vi "EnFlo_Tunnel_Display.vi"() -> ()   [LabVIEW 2013]
uses:
  <vilib>/gmath/NI_Gmath.lvlib
panel:
  out "Lateral profiles":cluster{"Y Axis Current":dbl[], dbl[]}[](graph)
  out "Setpoints":dbl[](array[numeric])
  in  "Subtract Setpoint?":bool
  out "Vert Disp (mm)  @ 14m":dbl
  out "Inlet St Dev":dbl format="%#.3g"
  out "Inlet mapping":dbl[][](graph)=[[0.00729, 0.18153463174730816, 0.17352738437348433, 1.6752433719500537, 8.231465735195274, 17.570357598383207, 23.099772817121426, 25.58386930448374, 25.31727725753219, 24.28926231541072, 18.717383219374323, 10.355253339797807, 2.7760273383248344, 0.3109897541921306, 0.08276881403435009, 0.06197], [0.04411, 0.1361526368018142, 0.04039202183336771, 1.5611636795339547, 8.176972694107874, 17.32000974741714, 24.257541358764026, 25.949153465972987, 26.01802540761648, 25.060373307424115, 18.284750328365213, 8.689831176707928, 2.642937641487066, 0.43219350072447926, -0.019957690739617468, 0.07351], [0.05478, 0.03446320268089581, 0.2086595806581808, 1.6919212249796047, 6.580368005180591, 14.333585185483123, 21.06810094963999, 23.709254571137723, 24.04768940379576, 21.01660820522005, 13.60443428327954, 6.2766496258038735, 1.7988963349022484, 0.2952877651784204, 0.05436788410934033, 0.1022], [0.04013, 0.06419557464541133, 0.2035068586120256, 1.3118741659450193, 4.7061387064566835, 9.009825946069038, 12.927700276268434, 17.003135081884164, 16.83885730812343, 12.902263313363814, 8.246161922417906, 4.035269404379355, 1.329605659745338, 0.24574055091433544, 0.012829784119986217, 0.08755], [0.04404, 0.022691144295571734, 0.19102098261858932, 0.8525411026079828, 2.2353542219792946, 3.966676465246214, 6.305347763088489, 8.17672908183636, 7.7348668140659, 5.703994479070454, 3.8329088824353237, 1.9256956625267279, 0.6611488869641811, 0.20508248283573002, 0.10119553469307395, 0.08441]]
  out "Floor Powers":cluster{"Array":dbl[], dbl[]}(graph)
  in  "Averaging time (mins)":dbl=0.5 format="%.2f"
  out "Ref_2":dbl format="%.3g"
  in  "History in Minutes":dbl
  out "Strat":cluster{dbl[], dbl[]}[](graph)
  out "Des Air Temp":dbl format="%#.2g"
  out "Heat Extraction kW":dbl format="%#.2g"
  out "Av Lab Temp":dbl format="%#.2g"
  out "Av Exit  Temp":dbl format="%#.2g"
  out "Exit Dem Temp":dbl format="%#.2g"
  out "Heat Exchanger Valve %":dbl format="%#.1f"
  out "Delta T":dbl format="%#.2g"
  out "Pump Speed %":dbl format="%#.0f"
  out "Meas Delta P":dbl format="%#.2g"
  out "Desired Delta P":dbl format="%#.2f"
  out "Return Pressure":dbl format="%#.2g"
  out "Supply Pressure":dbl format="%#.2g"
  out "Max Motor Temp":dbl format="%#.1g"
  out "% Speed Tweak":dbl format="%#.2g"
  out "Shaft RPM":dbl format="%#.2g"
  out "K Factor":dbl format="%#.2g"
  out "Tunnel Speed  m/s":dbl format="%.3g"
  out "Uni Chilled water Temp":dbl format="%#.2g"
  out "Mixing Valve %":dbl format="%#.1f"
  out "Dem Temp":dbl
  out "Return Temp":dbl format="%#.2g"
  out "Supply Temp":dbl format="%#.2g"
  out "Floor_Cooling:Enable":bool
  out "Chiller_Pump:Enable":bool
  out "Panel Temps":cluster{"Array":dbl[], dbl[]}[](graph)
  in  "Stop Button":bool
  out "Heaters Enabled":bool
  out "Inlet Heaters":cluster{"yi":dbl[], dbl[]}[](graph)
  # "Chiller Pump Information"
  # "Chilled Water"
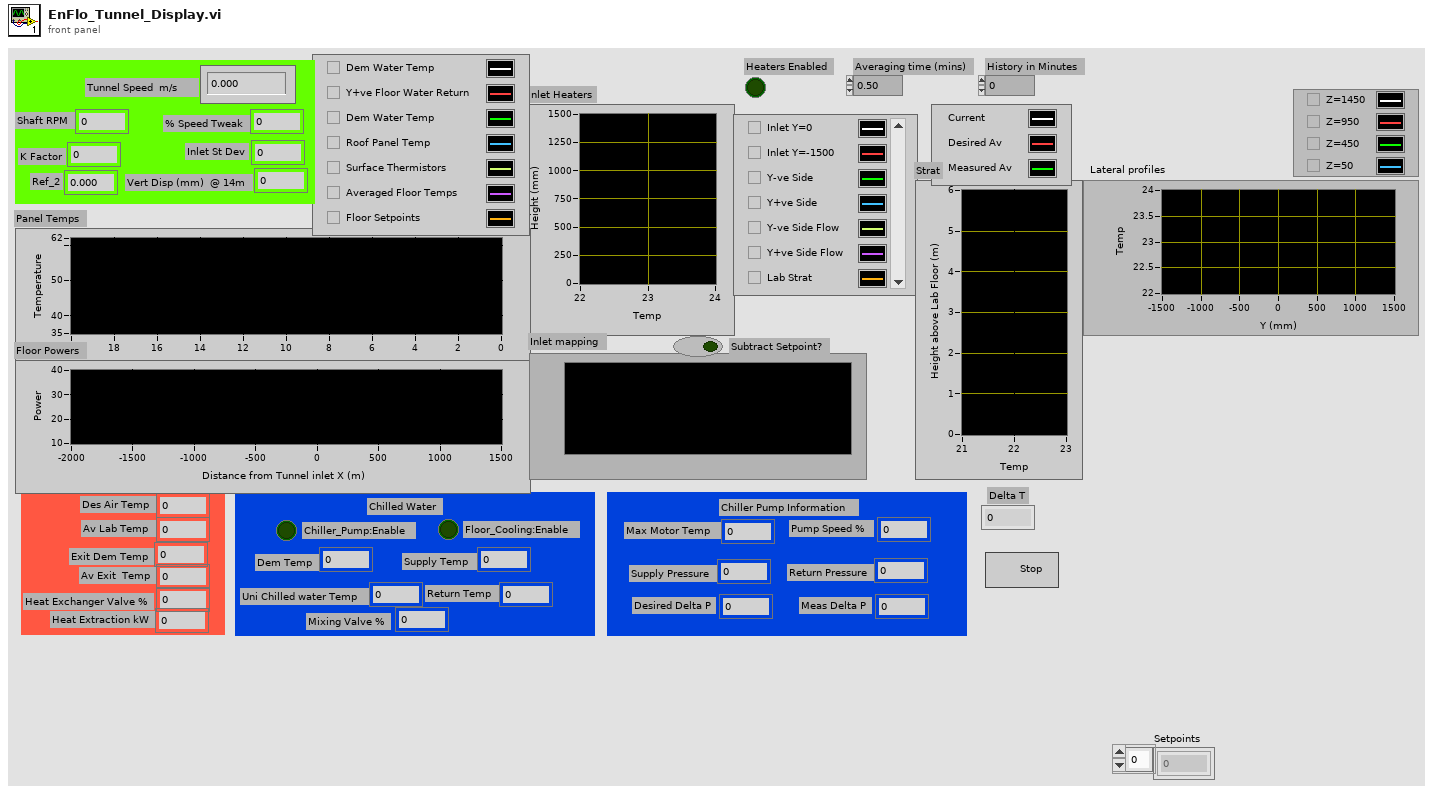
[diagram p1: front panel]
types:
  T1 = cluster{"X Max":dbl, "Y Max ":dbl, "X Scale":cluster{"Xo":dbl, "delta X":dbl}, "Y Scale":cluster{"Xo":dbl, "delta X":dbl}, "X Values":dbl[], "Y Values":dbl[], "Z Max":dbl, "Z Min":dbl}
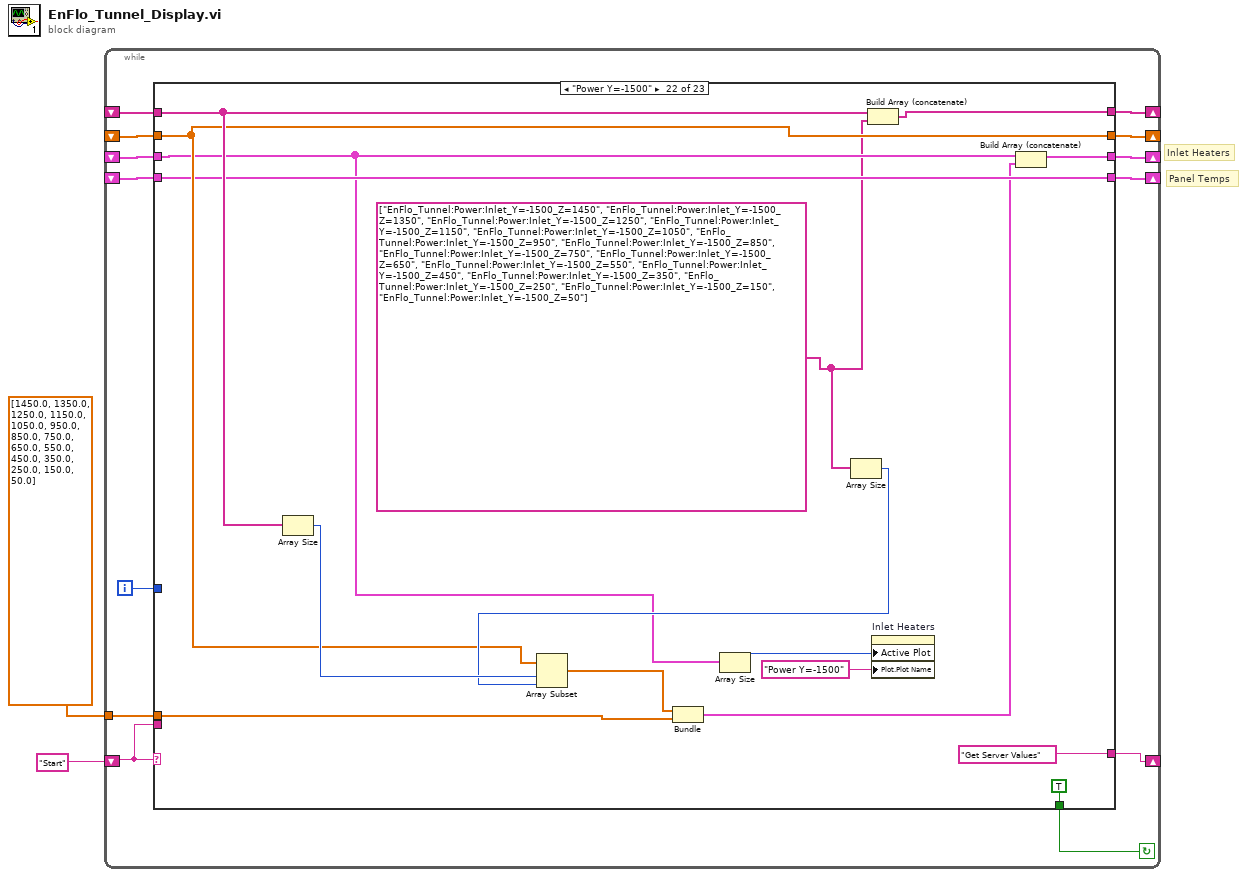
[diagram p0: block diagram]
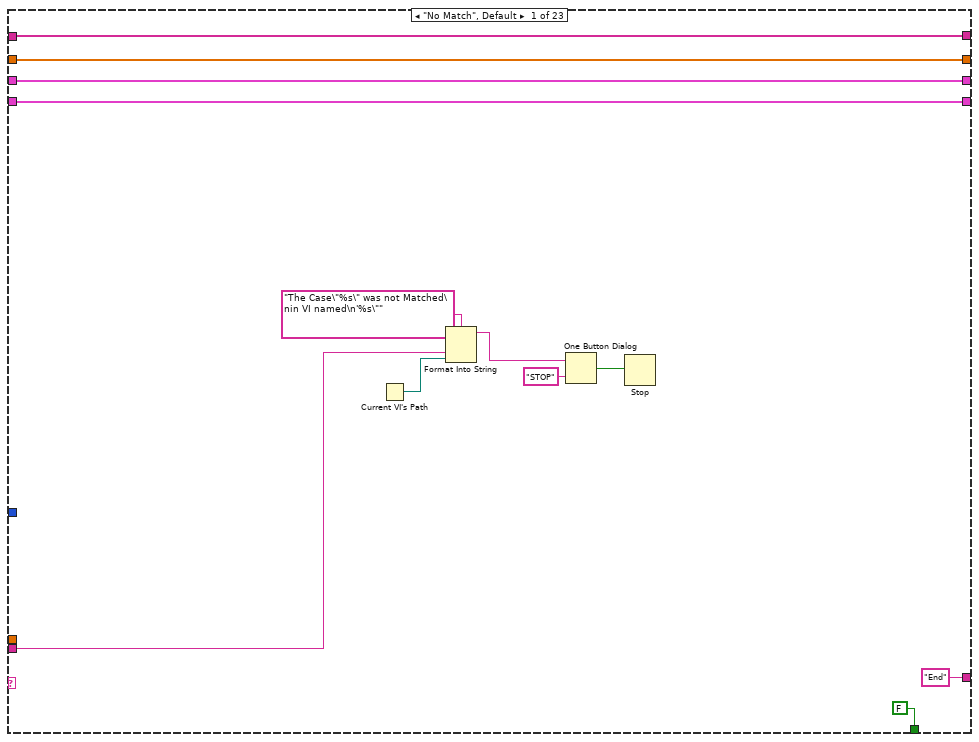
[diagram p2: hidden frame]
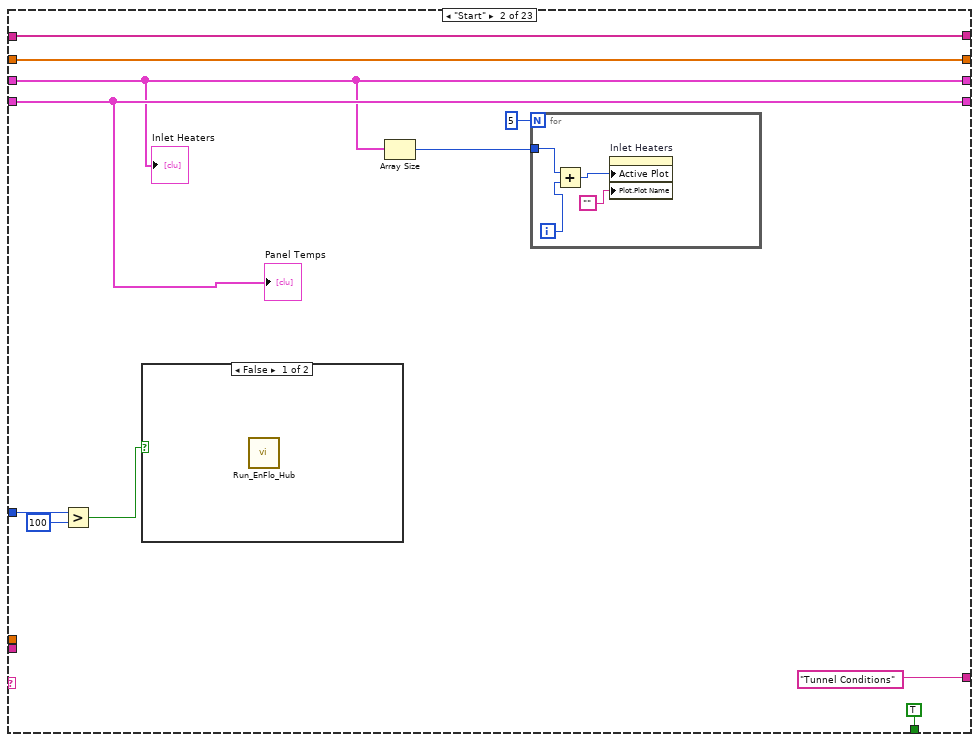
[diagram p3: hidden frame]
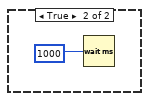
[diagram p4: hidden frame]
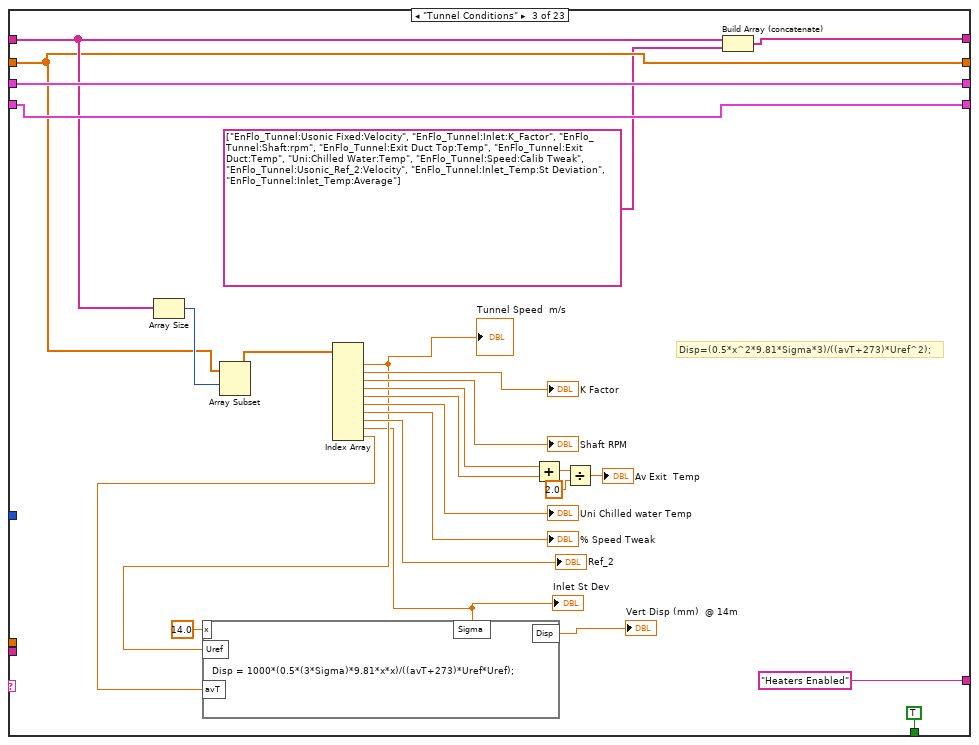
[diagram p5: hidden frame]
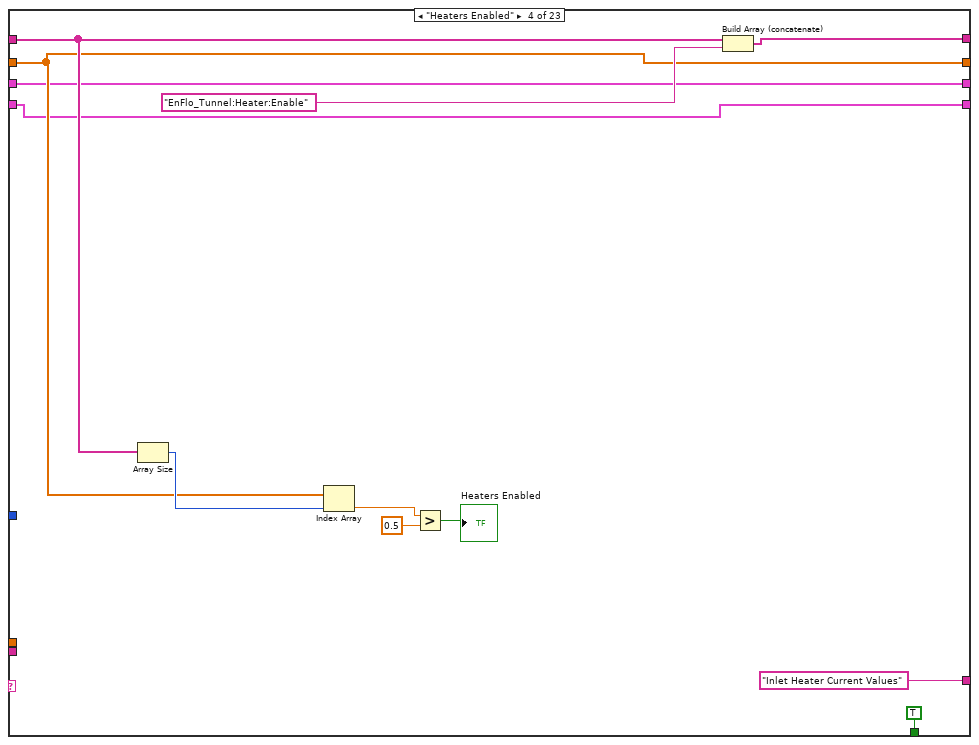
[diagram p6: hidden frame]
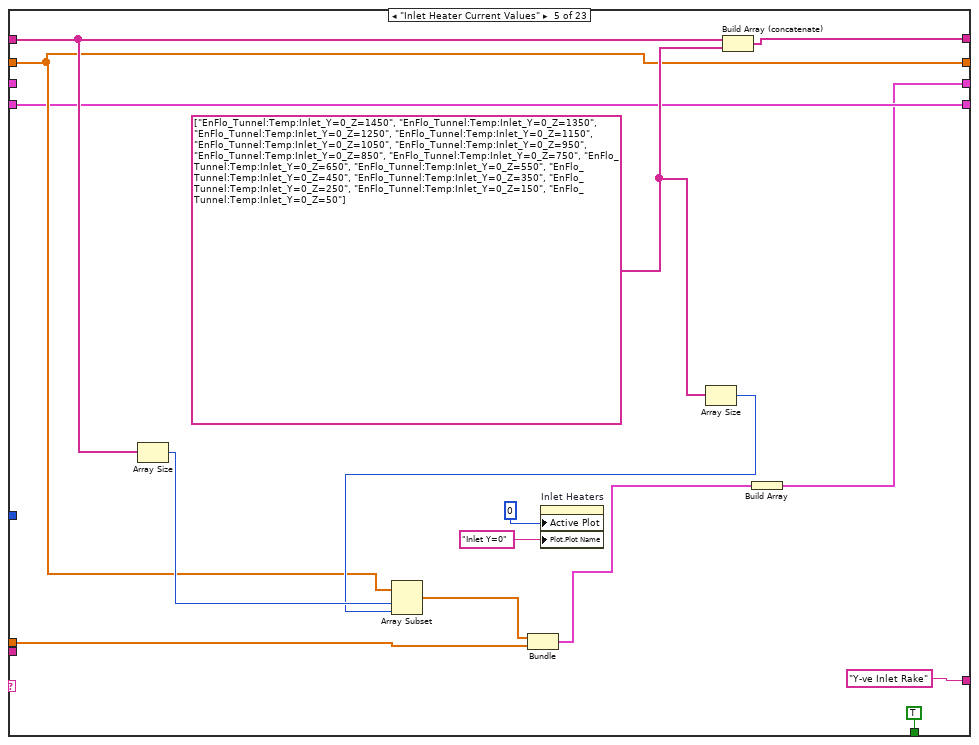
[diagram p7: hidden frame]
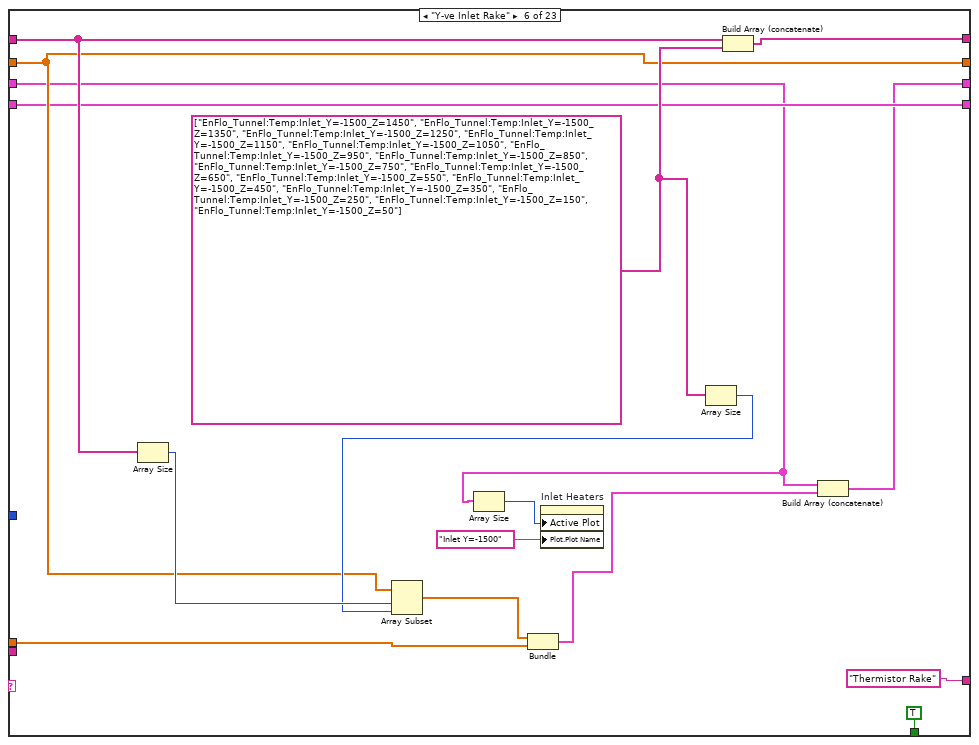
[diagram p8: hidden frame]
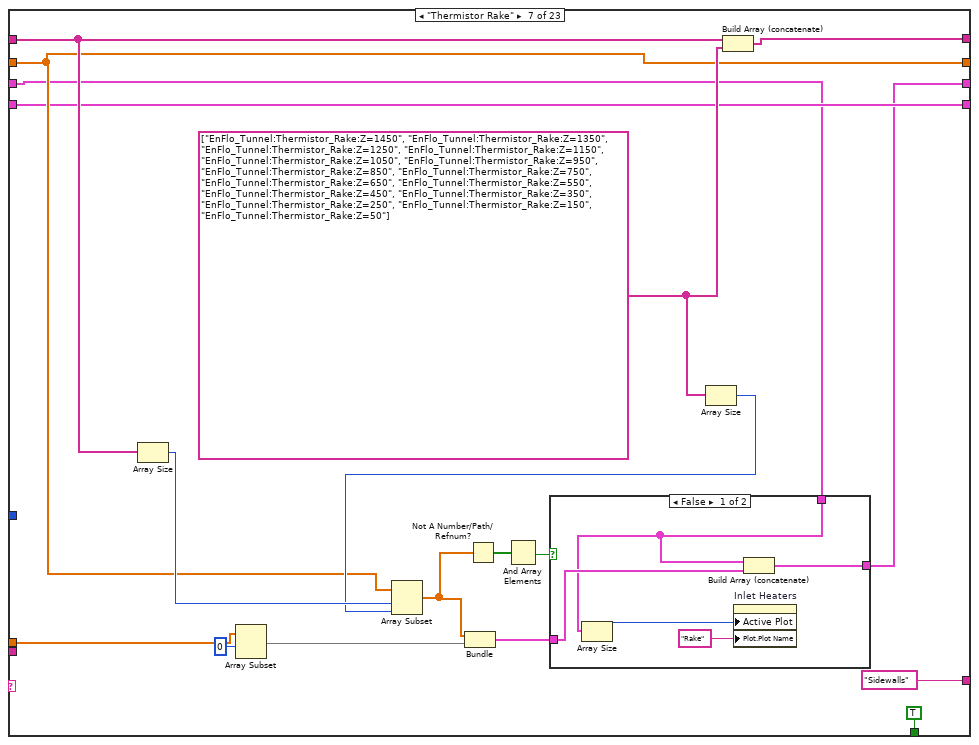
[diagram p9: hidden frame]
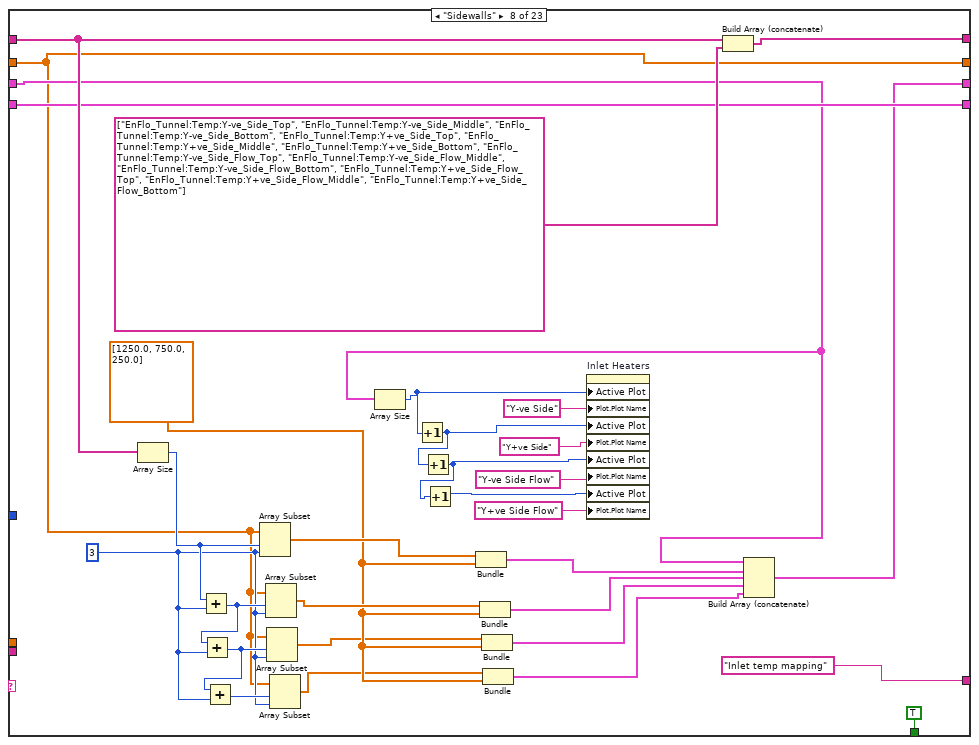
[diagram p11: hidden frame]
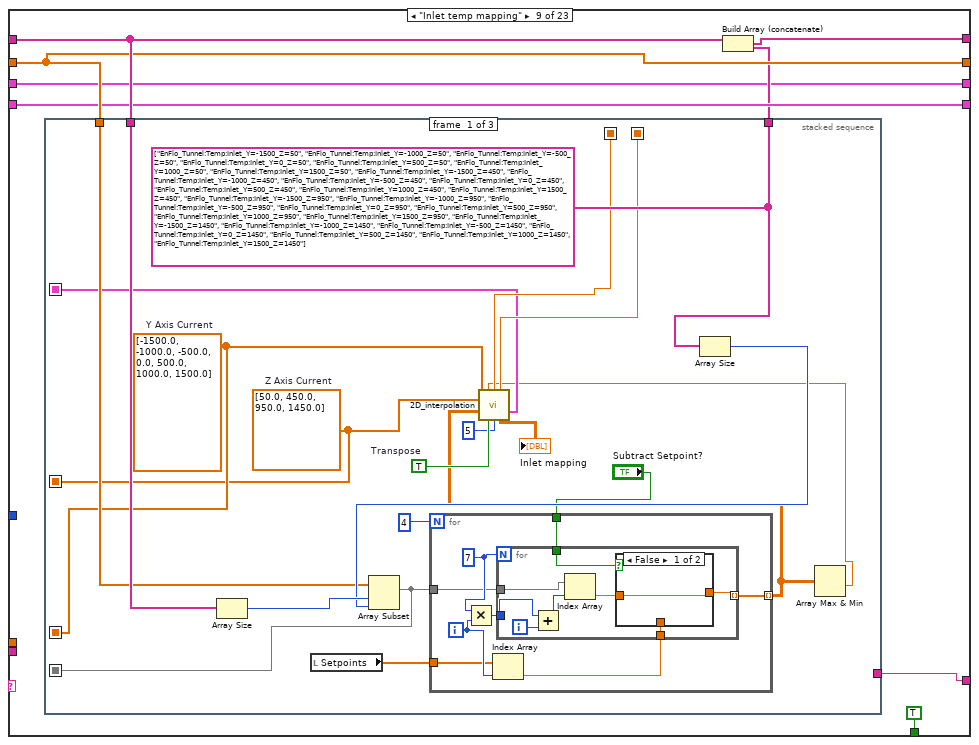
[diagram p12: hidden frame]
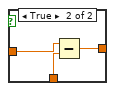
[diagram p13: hidden frame]
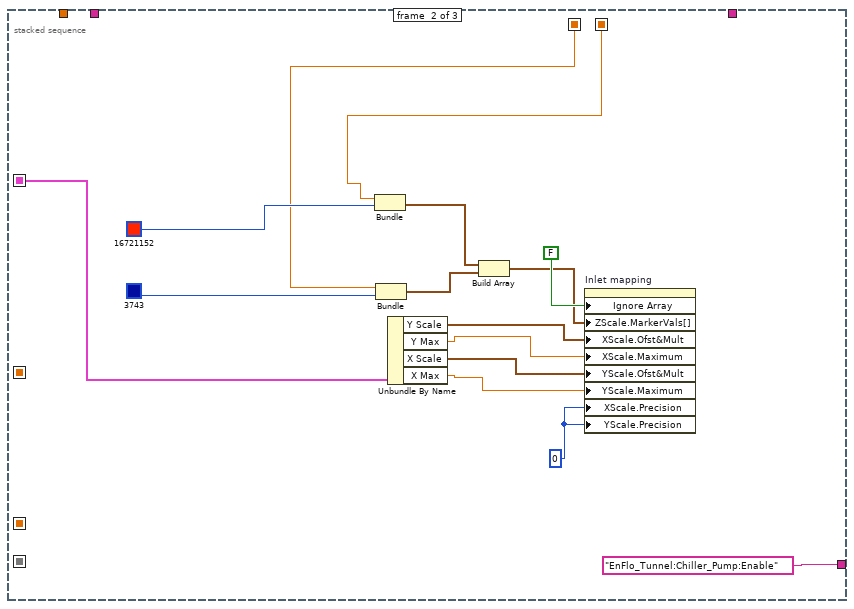
[diagram p14: hidden frame]
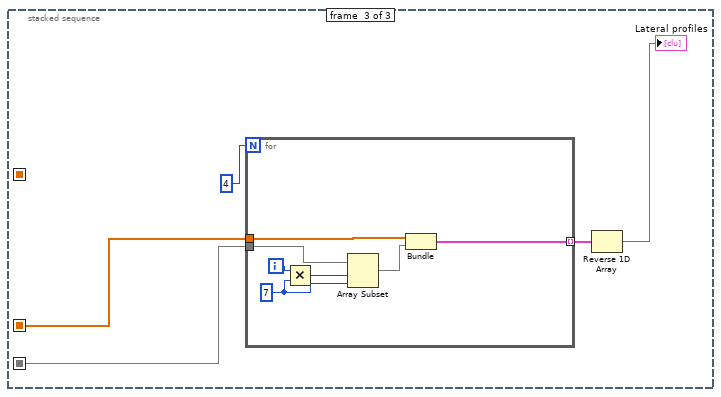
[diagram p15: hidden frame]
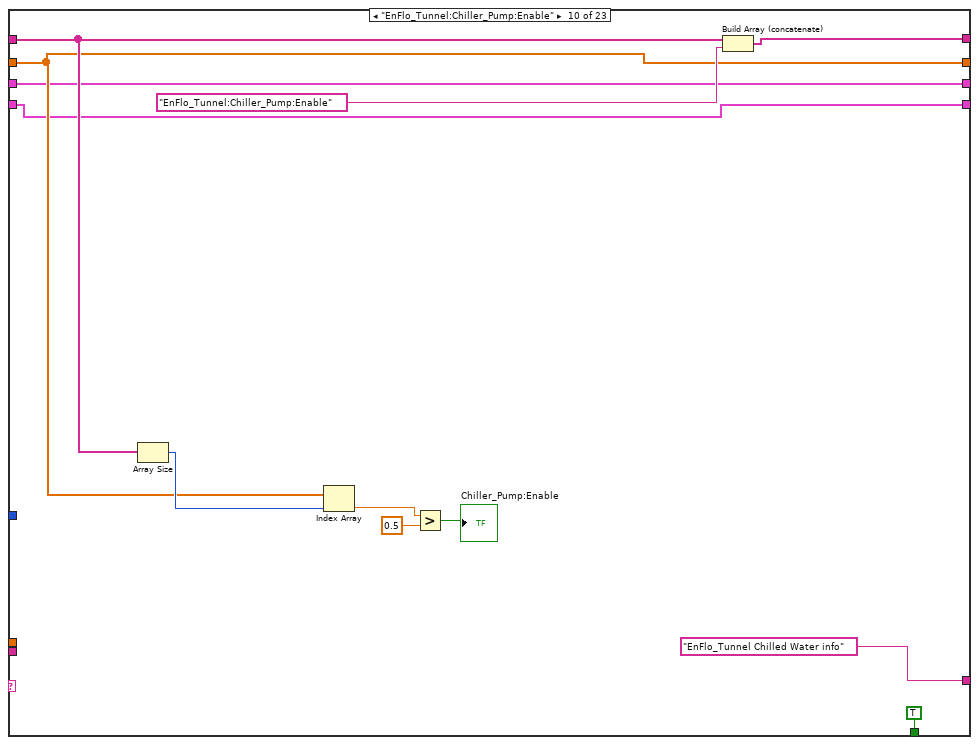
[diagram p16: hidden frame]
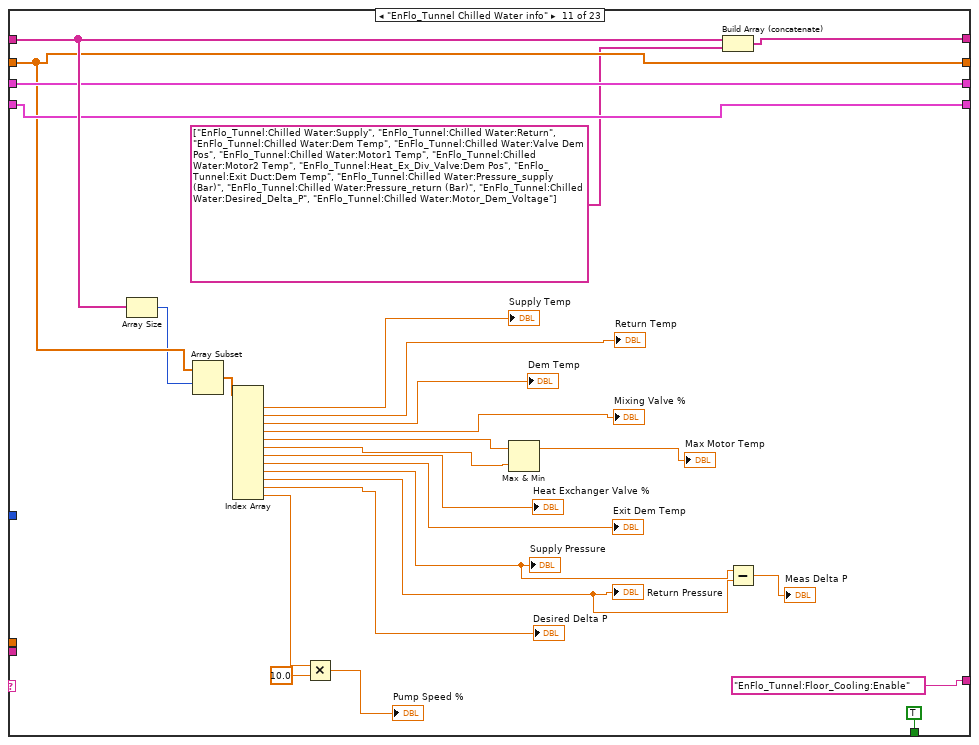
[diagram p17: hidden frame]
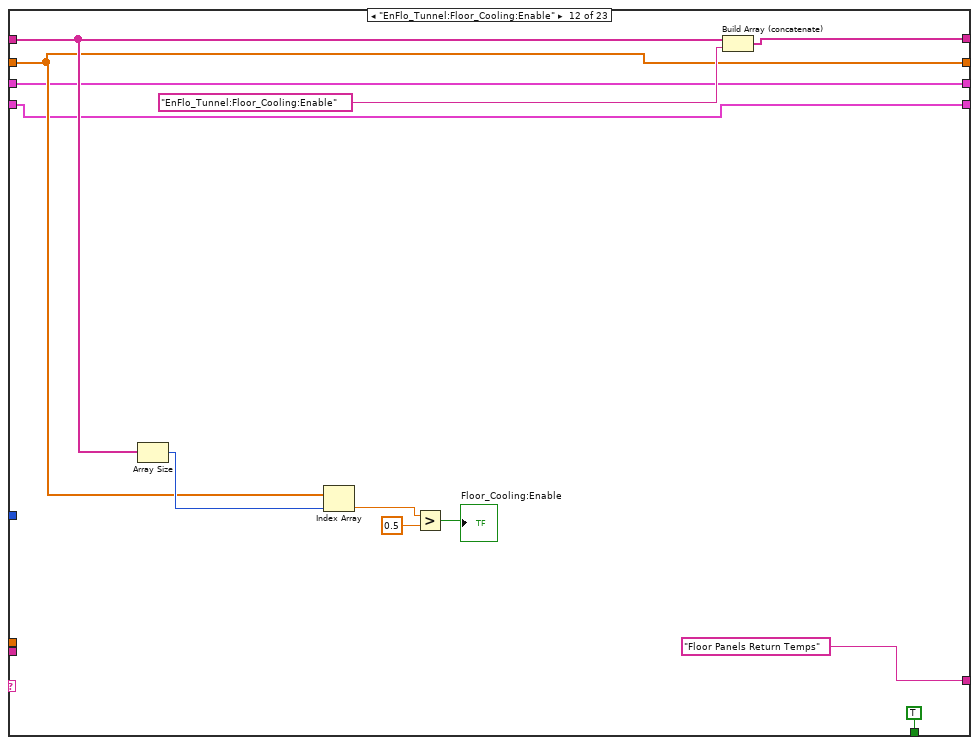
[diagram p18: hidden frame]
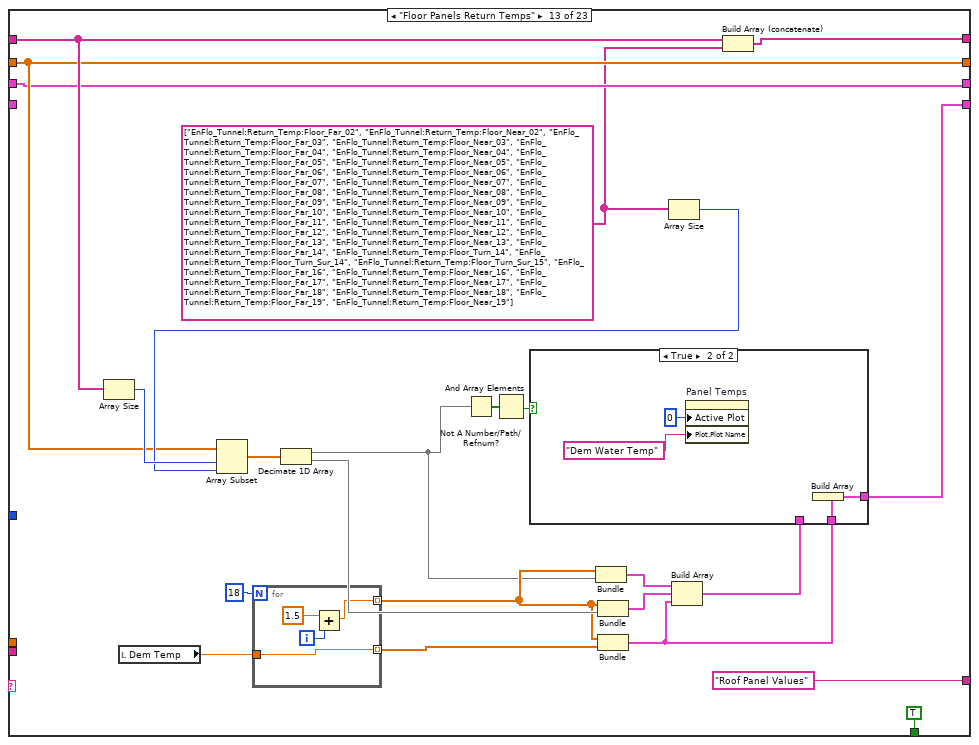
[diagram p19: hidden frame]
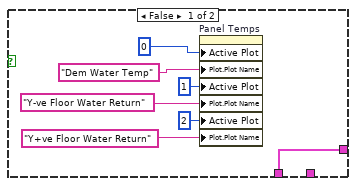
[diagram p20: hidden frame]
diagram:
  # "Panel Temps"
  # "Inlet Heaters"
  n1 = while {
    shift-right: [w13] -> _
    shift-left: "Start" -> [w14]
    shift-right: [w12] -> _
    shift-left: _ -> [w11]
    shift-right: [w9] -> _
    shift-left: _ -> [w10]
    shift-right: [w7] -> _
    shift-left: _ -> [w8]
    shift-right: [w6] -> _
    shift-left: _ -> [w5]
    tunnel: dbl[] [1450.0, 1350.0, 1250.0, 1150.0, 1050.0, 950.0, 850.0, 750.0, 650.0, 550.0, 450.0, 350.0, 250.0, 150.0, 50.0] -> [w3]
    i -> [w4]
    stop <- w15 continue-if-true
    n2 = case shown="\"Power Y=-1500\"" w14 {
      tunnel: [FALSE TRUE TRUE TRUE TRUE TRUE TRUE TRUE TRUE TRUE TRUE TRUE TRUE TRUE TRUE TRUE TRUE TRUE TRUE TRUE TRUE TRUE w500] -> w15
      tunnel: w14 -> [w21 _ _ _ _ _ _ _ _ _ _ _ _ _ _ _ _ _ _ _ _ _ _]
      tunnel: ["End" "Tunnel Conditions" "Heaters Enabled" "Inlet Heater Current Values" "Y-ve Inlet Rake" "Thermistor Rake" "Sidewalls" "Inlet temp mapping" w167 "EnFlo_Tunnel Chilled Water info" "EnFlo_Tunnel:Floor_Cooling:Enable" "Floor Panels Return Temps" "Roof Panel Values" "Floor Surface Panels" "Floor Panel Averages" "Floor Panel Setpoints" "Floor Panel Powers" "Lab Stratification" w398 "Inlet Heater Power Values" "Power Y=-1500" "Get Server Values" "Start"] -> w13
      tunnel: [w19 w37 w66 w78 w93 w109 w127 w164 w173 w251 w277 w289 w311 w340 w354 w368 w382 w395 w431 w456 w475 w491 string[] []] -> w12
      tunnel: w11 -> [w19 w37 w61 w77 w92 w108 w126 w163 w172 w250 w276 w288 w310 w339 w353 w367 w381 w394 w430 w455 w474 w490 w504]
      tunnel: w10 -> [w18 w36 w60 w74 w89 w105 w123 w138 w171 w247 w271 w285 w307 w336 w350 w364 w378 w391 w417 w452 w471 w487 _]
      tunnel: [w18 w36 w60 w74 w89 w105 w123 w138 w171 w247 w271 w285 w307 w336 w350 w364 w378 w391 w417 w452 w471 w487 w503] -> w9
      tunnel: w8 -> [w17 w30 w65 w73 _ w97 w119 w153 w168 w246 w275 w284 w305 w335 w349 w363 w377 w390 w400 w443 w463 w479 w498]
      tunnel: [w17 w30 w65 w73 w82 w100 w120 w159 w168 w246 w275 w284 w305 w335 w349 w363 w377 w390 w421 w450 w467 w483 w498] -> w7
      tunnel: w5 -> [w16 w34 w64 w69 w88 w104 w122 w162 w170 w242 w274 w280 _ w334 w348 w362 w376 w386 w429 w449 w469 w485 w497]
      tunnel: [w16 w34 w64 w69 w88 w104 w122 w162 w170 w242 w274 w280 w292 w333 w347 w361 w375 w386 w429 w449 w469 w485 w497] -> w6
      tunnel: w4 -> [_ w33 _ _ _ _ _ _ _ _ _ _ _ _ _ _ _ _ _ _ _ _ _]
      tunnel: w3 -> [_ _ _ _ w86 w102 w114 _ _ _ _ _ _ _ _ _ _ _ w403 w444 w468 w484 _]
      frame "No Match", Default {
        n3 = Current VI's Path() -> (path=w26:path)
        n4 = Format Into String(format string="The Case\"%s\" was not Matched\nin VI named\n'%s\"" ("Format String"), w21, w26) -> (resulting string=w23:string)  [unwired: 2 in, 1 out]
        n5 = One Button Dialog(message=w23, button name ("OK")="STOP") -> (true=w25:bool)
        n6 = Stop(stop? (T)=w25) -> ()
      }
      frame "Start" {
        n7 = Greater?(x=w33, y=100) -> (0:w31:bool)
        n8 = case shown="False" w31 {
          frame False {
            n9 = call "Run_EnFlo_Hub.vi"() -> ()  [unwired: 8 in]
          }
          frame True {
            n10 = Wait (ms)(milliseconds to wait=u32 1000 ("millisecond timer value")) -> ()  [unwired: 1 out]
          }
        }
        n11 = Array Size(array=w30) -> (size(s)=w28:i32)
        n12 = for {
          N: 5 -> [_]
          tunnel: w28 -> [w42]
          i -> [w41]
          n13 = Add(x=w42, y=w41) -> (x+y=w40:i32)
          n14 = property on="Inlet Heaters" class="XYGraph (strict)"("Active Plot"=w40, "Plot.Plot Name"="") -> ()  [unwired: 2 in, 2 out]
        }
        "Inlet Heaters" <- w30
        "Panel Temps" <- w34
      }
      frame "Tunnel Conditions" {
        # "Disp=(0.5*x^2*9.81*Sigma*3)/((avT+273)*Uref^2);"
        n15 = Array Size(array=w61) -> (size(s)=w63:i32)
        n16 = Array Subset(array=w60, index=w63) -> (w62:dbl[])  [unwired: 1 in]
        n17 = Index Array(array=w62) -> (element #1=w47:dbl, element #2=→"K Factor":dbl, element #3=→"Shaft RPM":dbl, element #4=w53:dbl, element #5=w52:dbl, element #6=→"Uni Chilled water Temp":dbl, element #7=→"% Speed Tweak":dbl, element #8=→"Ref_2":dbl, element #9=w46:dbl, element #10=w45:dbl)  [unwired: 10 in]
        "Tunnel Speed  m/s" <- w47
        "Inlet St Dev" <- w46
        n18 = formula code="Disp = 1000*(0.5*(3*Sigma)*9.81*x*x)/((avT+273)*Uref*Uref);"("x"=14.0 ("input variable"), "Uref"=w47, "Sigma"=w46, "avT"=w45) -> ("Disp"=→"Vert Disp (mm)  @ 14m":dbl)
        n19 = Add(x=w53, y=w52) -> (x+y=w57:dbl)
        n20 = Divide(x=w57, y=2.0) -> (x/y=→"Av Exit  Temp":dbl)
        n21 = Build Array (concatenate)(w61, string[] ["EnFlo_Tunnel:Usonic Fixed:Velocity", "EnFlo_Tunnel:Inlet:K_Factor", "EnFlo_Tunnel:Shaft:rpm", "EnFlo_Tunnel:Exit Duct Top:Temp", "EnFlo_Tunnel:Exit Duct:Temp", "Uni:Chilled Water:Temp", "EnFlo_Tunnel:Speed:Calib Tweak", "EnFlo_Tunnel:Usonic_Ref_2:Velocity", "EnFlo_Tunnel:Inlet_Temp:St Deviation", "EnFlo_Tunnel:Inlet_Temp:Average"] ("subarray")) -> (w66:string[])
      }
      frame "Heaters Enabled" {
        n22 = Array Size(array=w77) -> (size(s)=w75:i32)
        n23 = Index Array(array=w74, index=w75) -> (element=w72:dbl)
        n24 = Greater?(x=w72, y=0.5) -> (0:→"Heaters Enabled":bool)
        n25 = Build Array (concatenate)(w77, "EnFlo_Tunnel:Heater:Enable" ("Ch Name")) -> (w78:string[])
      }
      frame "Inlet Heater Current Values" {
        w94 = string[] ["EnFlo_Tunnel:Temp:Inlet_Y=0_Z=1450", "EnFlo_Tunnel:Temp:Inlet_Y=0_Z=1350", "EnFlo_Tunnel:Temp:Inlet_Y=0_Z=1250", "EnFlo_Tunnel:Temp:Inlet_Y=0_Z=1150", "EnFlo_Tunnel:Temp:Inlet_Y=0_Z=1050", "EnFlo_Tunnel:Temp:Inlet_Y=0_Z=950", "EnFlo_Tunnel:Temp:Inlet_Y=0_Z=850", "EnFlo_Tunnel:Temp:Inlet_Y=0_Z=750", "EnFlo_Tunnel:Temp:Inlet_Y=0_Z=650", "EnFlo_Tunnel:Temp:Inlet_Y=0_Z=550", "EnFlo_Tunnel:Temp:Inlet_Y=0_Z=450", "EnFlo_Tunnel:Temp:Inlet_Y=0_Z=350", "EnFlo_Tunnel:Temp:Inlet_Y=0_Z=250", "EnFlo_Tunnel:Temp:Inlet_Y=0_Z=150", "EnFlo_Tunnel:Temp:Inlet_Y=0_Z=50"] ("subarray")
        n26 = Array Size(array=w92) -> (size(s)=w91:i32)
        n27 = property on="Inlet Heaters" class="XYGraph (strict)"("Active Plot"=u32 0, "Plot.Plot Name"="Inlet Y=0") -> ()  [unwired: 2 in, 2 out]
        n28 = Array Size(array=w94) -> (size(s)=w90:i32)
        n29 = Array Subset(array=w89, index=w91, length=w90) -> (w87:dbl[])
        n30 = Bundle(w87, w86) -> (w83:cluster{dbl[], dbl[]})  [unwired: 1 in]
        n31 = Build Array (concatenate)(w92, w94) -> (w93:string[])
        n32 = Build Array(w83) -> (w82:cluster{dbl[], dbl[]}[])
      }
      frame "Y-ve Inlet Rake" {
        w110 = string[] ["EnFlo_Tunnel:Temp:Inlet_Y=-1500_Z=1450", "EnFlo_Tunnel:Temp:Inlet_Y=-1500_Z=1350", "EnFlo_Tunnel:Temp:Inlet_Y=-1500_Z=1250", "EnFlo_Tunnel:Temp:Inlet_Y=-1500_Z=1150", "EnFlo_Tunnel:Temp:Inlet_Y=-1500_Z=1050", "EnFlo_Tunnel:Temp:Inlet_Y=-1500_Z=950", "EnFlo_Tunnel:Temp:Inlet_Y=-1500_Z=850", "EnFlo_Tunnel:Temp:Inlet_Y=-1500_Z=750", "EnFlo_Tunnel:Temp:Inlet_Y=-1500_Z=650", "EnFlo_Tunnel:Temp:Inlet_Y=-1500_Z=550", "EnFlo_Tunnel:Temp:Inlet_Y=-1500_Z=450", "EnFlo_Tunnel:Temp:Inlet_Y=-1500_Z=350", "EnFlo_Tunnel:Temp:Inlet_Y=-1500_Z=250", "EnFlo_Tunnel:Temp:Inlet_Y=-1500_Z=150", "EnFlo_Tunnel:Temp:Inlet_Y=-1500_Z=50"] ("subarray")
        n33 = Array Size(array=w108) -> (size(s)=w107:i32)
        n34 = Array Size(array=w97) -> (size(s)=w96:i32)
        n35 = property on="Inlet Heaters" class="XYGraph (strict)"("Active Plot"=w96, "Plot.Plot Name"="Inlet Y=-1500") -> ()  [unwired: 2 in, 2 out]
        n36 = Array Size(array=w110) -> (size(s)=w106:i32)
        n37 = Array Subset(array=w105, index=w107, length=w106) -> (w103:dbl[])
        n38 = Bundle(w103, w102) -> (w98:cluster{dbl[], dbl[]})  [unwired: 1 in]
        n39 = Build Array (concatenate)(w108, w110) -> (w109:string[])
        n40 = Build Array (concatenate)(w97, w98) -> (w100:cluster{"yi":dbl[], dbl[]}[])
      }
      frame "Thermistor Rake" {
        w128 = string[] ["EnFlo_Tunnel:Thermistor_Rake:Z=1450", "EnFlo_Tunnel:Thermistor_Rake:Z=1350", "EnFlo_Tunnel:Thermistor_Rake:Z=1250", "EnFlo_Tunnel:Thermistor_Rake:Z=1150", "EnFlo_Tunnel:Thermistor_Rake:Z=1050", "EnFlo_Tunnel:Thermistor_Rake:Z=950", "EnFlo_Tunnel:Thermistor_Rake:Z=850", "EnFlo_Tunnel:Thermistor_Rake:Z=750", "EnFlo_Tunnel:Thermistor_Rake:Z=650", "EnFlo_Tunnel:Thermistor_Rake:Z=550", "EnFlo_Tunnel:Thermistor_Rake:Z=450", "EnFlo_Tunnel:Thermistor_Rake:Z=350", "EnFlo_Tunnel:Thermistor_Rake:Z=250", "EnFlo_Tunnel:Thermistor_Rake:Z=150", "EnFlo_Tunnel:Thermistor_Rake:Z=50"] ("subarray")
        n41 = Array Size(array=w126) -> (size(s)=w125:i32)
        n42 = Array Subset(array=w114, index=0) -> (w112:dbl[])  [unwired: 1 in]
        n43 = Array Size(array=w128) -> (size(s)=w124:i32)
        n44 = Array Subset(array=w123, index=w125, length=w124) -> (w118:dbl[])
        n45 = Bundle(w118, w112) -> (w115:cluster{dbl[], dbl[]})  [unwired: 1 in]
        n46 = Not A Number/Path/Refnum?(number/path/refnum=w118) -> (NaN/Path/Refnum?=w117:bool[])
        n47 = And Array Elements(Boolean array=w117) -> (logical AND=w116:bool)
        n48 = case shown="False" w116 {
          tunnel: [w134 w135] -> w120
          tunnel: w119 -> [w130 w135]
          tunnel: w115 -> [w133 _]
          frame False {
            n49 = Array Size(array=w130) -> (size(s)=w131:i32)
            n50 = property on="Inlet Heaters" class="XYGraph (strict)"("Active Plot"=w131, "Plot.Plot Name"="Rake") -> ()  [unwired: 2 in, 2 out]
            n51 = Build Array (concatenate)(w130, w133) -> (w134:cluster{"yi":dbl[], dbl[]}[])
          }
          frame True {
          }
        }
        n52 = Build Array (concatenate)(w126, w128) -> (w127:string[])
      }
      frame "Sidewalls" {
        w141 = dbl[] [1250.0, 750.0, 250.0]
        w142 = 3 ("length")
        n53 = Array Size(array=w163) -> (size(s)=w158:i32)
        n54 = Add(x=w158, y=w142) -> (x+y=w144:i32)
        n55 = Add(x=w144, y=w142) -> (x+y=w143:i32)
        n56 = Add(x=w143, y=w142) -> (x+y=w145:i32)
        n57 = Array Subset(array=w138, index=w158, length=w142) -> (w157:dbl[])
        n58 = Array Subset(array=w138, index=w144, length=w142) -> (w156:dbl[])
        n59 = Array Subset(array=w138, index=w143, length=w142) -> (w140:dbl[])
        n60 = Array Subset(array=w138, index=w145, length=w142) -> (w139:dbl[])
        n61 = Array Size(array=w153) -> (size(s)=w151:i32)
        n62 = Increment(x=w151) -> (x+1=w148:i32)
        n63 = Increment(x=w148) -> (x+1=w146:i32)
        n64 = Increment(x=w146) -> (x+1=w147:i32)
        n65 = Bundle(w157, w141) -> (w160:cluster{dbl[], dbl[]})  [unwired: 1 in]
        n66 = Bundle(w156, w141) -> (w155:cluster{dbl[], dbl[]})  [unwired: 1 in]
        n67 = Bundle(w140, w141) -> (w137:cluster{dbl[], dbl[]})  [unwired: 1 in]
        n68 = Bundle(w139, w141) -> (w136:cluster{dbl[], dbl[]})  [unwired: 1 in]
        n69 = property on="Inlet Heaters" class="XYGraph (strict)"("Active Plot"=w151, "Plot.Plot Name"="Y-ve Side", "Active Plot"=w148, "Plot.Plot Name"="Y+ve Side", "Active Plot"=w146, "Plot.Plot Name"="Y-ve Side Flow", "Active Plot"=w147, "Plot.Plot Name"="Y+ve Side Flow") -> ()  [unwired: 2 in, 2 out]
        n70 = Build Array (concatenate)(w163, string[] ["EnFlo_Tunnel:Temp:Y-ve_Side_Top", "EnFlo_Tunnel:Temp:Y-ve_Side_Middle", "EnFlo_Tunnel:Temp:Y-ve_Side_Bottom", "EnFlo_Tunnel:Temp:Y+ve_Side_Top", "EnFlo_Tunnel:Temp:Y+ve_Side_Middle", "EnFlo_Tunnel:Temp:Y+ve_Side_Bottom", "EnFlo_Tunnel:Temp:Y-ve_Side_Flow_Top", "EnFlo_Tunnel:Temp:Y-ve_Side_Flow_Middle", "EnFlo_Tunnel:Temp:Y-ve_Side_Flow_Bottom", "EnFlo_Tunnel:Temp:Y+ve_Side_Flow_Top", "EnFlo_Tunnel:Temp:Y+ve_Side_Flow_Middle", "EnFlo_Tunnel:Temp:Y+ve_Side_Flow_Bottom"] ("subarray")) -> (w164:string[])
        n71 = Build Array (concatenate)(w153, w160, w155, w137, w136) -> (w159:cluster{"yi":dbl[], dbl[]}[])
      }
      frame "Inlet temp mapping" {
        n72 = stacked-sequence {
          seq-local: [w185 _ _] -> [_ w222 _]
          seq-local: [w184 _ _] -> [_ w223 _]
          seq-local: [w183 _ _] -> [_ w218 _]
          seq-local: [w177 _ _] -> [_ _ w232]
          seq-local: [w176 _ _] -> [_ _ w233]
          seq-local: [w175 _ _] -> [_ _ _]
          tunnel: w172 -> [w193 _ _]
          tunnel: w171 -> [w190 _ _]
          tunnel: [w189 _ _] -> w169
          tunnel: [_ "EnFlo_Tunnel:Chiller_Pump:Enable" _] -> w167
          frame #0 {
            w187 = TRUE  # Transpose
            w175 = dbl[] [50.0, 450.0, 950.0, 1450.0]  # Z Axis Current
            w176 = dbl[] [-1500.0, -1000.0, -500.0, 0.0, 500.0, 1000.0, 1500.0]  # Y Axis Current
            w189 = string[] ["EnFlo_Tunnel:Temp:Inlet_Y=-1500_Z=50", "EnFlo_Tunnel:Temp:Inlet_Y=-1000_Z=50", "EnFlo_Tunnel:Temp:Inlet_Y=-500_Z=50", "EnFlo_Tunnel:Temp:Inlet_Y=0_Z=50", "EnFlo_Tunnel:Temp:Inlet_Y=500_Z=50", "EnFlo_Tunnel:Temp:Inlet_Y=1000_Z=50", "EnFlo_Tunnel:Temp:Inlet_Y=1500_Z=50", "EnFlo_Tunnel:Temp:Inlet_Y=-1500_Z=450", "EnFlo_Tunnel:Temp:Inlet_Y=-1000_Z=450", "EnFlo_Tunnel:Temp:Inlet_Y=-500_Z=450", "EnFlo_Tunnel:Temp:Inlet_Y=0_Z=450", "EnFlo_Tunnel:Temp:Inlet_Y=500_Z=450", "EnFlo_Tunnel:Temp:Inlet_Y=1000_Z=450", "EnFlo_Tunnel:Temp:Inlet_Y=1500_Z=450", "EnFlo_Tunnel:Temp:Inlet_Y=-1500_Z=950", "EnFlo_Tunnel:Temp:Inlet_Y=-1000_Z=950", "EnFlo_Tunnel:Temp:Inlet_Y=-500_Z=950", "EnFlo_Tunnel:Temp:Inlet_Y=0_Z=950", "EnFlo_Tunnel:Temp:Inlet_Y=500_Z=950", "EnFlo_Tunnel:Temp:Inlet_Y=1000_Z=950", "EnFlo_Tunnel:Temp:Inlet_Y=1500_Z=950", "EnFlo_Tunnel:Temp:Inlet_Y=-1500_Z=1450", "EnFlo_Tunnel:Temp:Inlet_Y=-1000_Z=1450", "EnFlo_Tunnel:Temp:Inlet_Y=-500_Z=1450", "EnFlo_Tunnel:Temp:Inlet_Y=0_Z=1450", "EnFlo_Tunnel:Temp:Inlet_Y=500_Z=1450", "EnFlo_Tunnel:Temp:Inlet_Y=1000_Z=1450", "EnFlo_Tunnel:Temp:Inlet_Y=1500_Z=1450"] ("subarray")
            n73 = Array Size(array=w193) -> (size(s)=w192:i32)
            n74 = local read "Setpoints"() -> (w181:dbl[])
            n75 = Array Size(array=w189) -> (size(s)=w191:i32)
            n76 = Array Subset(array=w190, index=w192, length=w191) -> (w177:dbl[])
            n77 = for {
              N: 4 -> [_]
              tunnel: [w199] -> w179 mode=indexing
              tunnel: w181 -> [w197]
              tunnel: "Subtract Setpoint?" -> [w196]
              tunnel: w177 -> [w194]
              i -> [w198]
              w201 = 7
              n78 = Multiply(x=w201, y=w198) -> (x*y=w200:i32)
              n79 = Index Array(array=w197, index=w198) -> (element=w195:dbl)
              n80 = for {
                N: w201 -> [_]
                tunnel: w200 -> [w208]
                tunnel: w194 -> [w206]
                tunnel: [w202] -> w199 mode=indexing
                tunnel: w196 -> [w205]
                tunnel: w195 -> [w203]
                i -> [w209]
                n81 = Add(x=w208, y=w209) -> (x+y=w207:i32)
                n82 = Index Array(array=w206, index=w207) -> (element=w204:dbl)
                n83 = case shown="False" w205 {
                  tunnel: w204 -> [w210 w213]
                  tunnel: w203 -> [_ w212]
                  tunnel: [w210 w211] -> w202
                  frame False {
                  }
                  frame True {
                    n84 = Subtract(x=w213, y=w212) -> (x-y=w211:dbl)
                  }
                }
              }
            }
            n85 = Array Max & Min(array=w179) -> (min value=w178:dbl)  [unwired: 3 out]
            n86 = call "2D_interpolation.vi"("X Axis Current"=w176, "Min Z Value In"=w178, "Y axis Current"=w175, "Plot In"=w179, "Transpose"=w187, "Point Size"=5) -> ("min Z value"=w185:dbl, "max Z value"=w184:dbl, "Axis info"=w183:T1, "Plot Out"=→"Inlet mapping":dbl[][])  [unwired: 2 in, 4 out]
          }
          frame #1 {
            w219 = u8 0 ("X Scale.Display Format:Precision")
            n87 = Bundle("max Z value"=w223, u32 16721152) -> (w226:cluster{"max Z value":dbl, u32})  [unwired: 1 out]
            n88 = Bundle("min Z value"=w222, u32 3743) -> (w227:cluster{"min Z value":dbl, u32})  [unwired: 1 out]
            n89 = Unbundle By Name(w218) -> ("Y Scale"=w217:cluster{"Xo":dbl, "delta X":dbl}, "Y Max"=w216:dbl, "X Scale"=w215:cluster{"Xo":dbl, "delta X":dbl}, "X Max"=w214:dbl)
            n90 = Build Array(w226, w227) -> (w220:cluster{"min Z value":dbl, u32}[])
            n91 = property on="Inlet mapping" class="IntGraph (strict)"("Ignore Array"=FALSE, "ZScale.MarkerVals[]"=w220, "XScale.Ofst&Mult"=w217, "XScale.Maximum"=w216, "YScale.Ofst&Mult"=w215, "YScale.Maximum"=w214, "XScale.Precision"=w219, "YScale.Precision"=w219) -> ()  [unwired: 2 in, 2 out]
          }
          frame #2 {
            n92 = for {
              N: 4 -> [_]
              tunnel: w233 -> [w240]
              tunnel: w232 -> [w239]
              tunnel: [w234] -> w230 mode=indexing
              i -> [w236]
              w238 = 7 ("length")
              n93 = Multiply(x=w236, y=w238) -> (x*y=w237:i32)
              n94 = Array Subset(array=w239, index=w237, length=w238) -> (w235:dbl[])
              n95 = Bundle("Y Axis Current"=w240, w235) -> (w234:cluster{"Y Axis Current":dbl[], dbl[]})  [unwired: 1 in]
            }
            n96 = Reverse 1D Array(array=w230) -> (reversed array=→"Lateral profiles":cluster{"Y Axis Current":dbl[], dbl[]}[])
          }
        }
        n97 = Build Array (concatenate)(w172, w169) -> (w173:string[])
      }
      frame "EnFlo_Tunnel:Chiller_Pump:Enable" {
        n98 = Array Size(array=w250) -> (size(s)=w248:i32)
        n99 = Index Array(array=w247, index=w248) -> (element=w245:dbl)
        n100 = Greater?(x=w245, y=0.5) -> (0:→"Chiller_Pump:Enable":bool)
        n101 = Build Array (concatenate)(w250, "EnFlo_Tunnel:Chiller_Pump:Enable" ("Ch Name")) -> (w251:string[])
      }
      frame "EnFlo_Tunnel Chilled Water info" {
        n102 = Array Size(array=w276) -> (size(s)=w270:i32)
        n103 = Array Subset(array=w271, index=w270) -> (w269:dbl[])  [unwired: 1 in]
        n104 = Index Array(array=w269) -> (element #1=→"Supply Temp":dbl, element #2=→"Return Temp":dbl, element #3=→"Dem Temp":dbl, element #4=→"Mixing Valve %":dbl, element #5=w256:dbl, element #6=w255:dbl, element #7=→"Heat Exchanger Valve %":dbl, element #8=→"Exit Dem Temp":dbl, element #9=w261:dbl, element #10=w260:dbl, element #11=→"Desired Delta P":dbl, element #12=w253:dbl)  [unwired: 12 in]
        "Supply Pressure" <- w261
        "Return Pressure" <- w260
        n105 = Multiply(x=w253, y=10.0) -> (x*y=→"Pump Speed %":dbl)
        n106 = Max & Min(x=w256, y=w255) -> (max(x,y)=→"Max Motor Temp":dbl)  [unwired: 1 out]
        n107 = Build Array (concatenate)(w276, string[] ["EnFlo_Tunnel:Chilled Water:Supply", "EnFlo_Tunnel:Chilled Water:Return", "EnFlo_Tunnel:Chilled Water:Dem Temp", "EnFlo_Tunnel:Chilled Water:Valve Dem Pos", "EnFlo_Tunnel:Chilled Water:Motor1 Temp", "EnFlo_Tunnel:Chilled Water:Motor2 Temp", "EnFlo_Tunnel:Heat_Ex_Div_Valve:Dem Pos", "EnFlo_Tunnel:Exit Duct:Dem Temp", "EnFlo_Tunnel:Chilled Water:Pressure_supply (Bar)", "EnFlo_Tunnel:Chilled Water:Pressure_return (Bar)", "EnFlo_Tunnel:Chilled Water:Desired_Delta_P", "EnFlo_Tunnel:Chilled Water:Motor_Dem_Voltage"] ("subarray")) -> (w277:string[])
        n108 = Subtract(x=w261, y=w260) -> (x-y=→"Meas Delta P":dbl)
      }
      frame "EnFlo_Tunnel:Floor_Cooling:Enable" {
        n109 = Array Size(array=w288) -> (size(s)=w286:i32)
        n110 = Index Array(array=w285, index=w286) -> (element=w283:dbl)
        n111 = Greater?(x=w283, y=0.5) -> (0:→"Floor_Cooling:Enable":bool)
        n112 = Build Array (concatenate)(w288, "EnFlo_Tunnel:Floor_Cooling:Enable" ("Ch Name")) -> (w289:string[])
      }
      frame "Floor Panels Return Temps" {
        w304 = string[] ["EnFlo_Tunnel:Return_Temp:Floor_Far_02", "EnFlo_Tunnel:Return_Temp:Floor_Near_02", "EnFlo_Tunnel:Return_Temp:Floor_Far_03", "EnFlo_Tunnel:Return_Temp:Floor_Near_03", "EnFlo_Tunnel:Return_Temp:Floor_Far_04", "EnFlo_Tunnel:Return_Temp:Floor_Near_04", "EnFlo_Tunnel:Return_Temp:Floor_Far_05", "EnFlo_Tunnel:Return_Temp:Floor_Near_05", "EnFlo_Tunnel:Return_Temp:Floor_Far_06", "EnFlo_Tunnel:Return_Temp:Floor_Near_06", "EnFlo_Tunnel:Return_Temp:Floor_Far_07", "EnFlo_Tunnel:Return_Temp:Floor_Near_07", "EnFlo_Tunnel:Return_Temp:Floor_Far_08", "EnFlo_Tunnel:Return_Temp:Floor_Near_08", "EnFlo_Tunnel:Return_Temp:Floor_Far_09", "EnFlo_Tunnel:Return_Temp:Floor_Near_09", "EnFlo_Tunnel:Return_Temp:Floor_Far_10", "EnFlo_Tunnel:Return_Temp:Floor_Near_10", "EnFlo_Tunnel:Return_Temp:Floor_Far_11", "EnFlo_Tunnel:Return_Temp:Floor_Near_11", "EnFlo_Tunnel:Return_Temp:Floor_Far_12", "EnFlo_Tunnel:Return_Temp:Floor_Near_12", "EnFlo_Tunnel:Return_Temp:Floor_Far_13", "EnFlo_Tunnel:Return_Temp:Floor_Near_13", "EnFlo_Tunnel:Return_Temp:Floor_Far_14", "EnFlo_Tunnel:Return_Temp:Floor_Turn_14", "EnFlo_Tunnel:Return_Temp:Floor_Turn_Sur_14", "EnFlo_Tunnel:Return_Temp:Floor_Turn_Sur_15", "EnFlo_Tunnel:Return_Temp:Floor_Far_16", "EnFlo_Tunnel:Return_Temp:Floor_Near_16", "EnFlo_Tunnel:Return_Temp:Floor_Far_17", "EnFlo_Tunnel:Return_Temp:Floor_Near_17", "EnFlo_Tunnel:Return_Temp:Floor_Far_18", "EnFlo_Tunnel:Return_Temp:Floor_Near_18", "EnFlo_Tunnel:Return_Temp:Floor_Far_19", "EnFlo_Tunnel:Return_Temp:Floor_Near_19"] ("subarray")
        n113 = Array Size(array=w310) -> (size(s)=w309:i32)
        n114 = local read "Dem Temp"() -> (w298:dbl)
        n115 = for {
          N: 18 -> [_]
          tunnel: [w327] -> w299 mode=indexing
          tunnel: w298 -> [w325]
          tunnel: [w325] -> w297 mode=indexing
          i -> [w328]
          n116 = Add(x=1.5, y=w328) -> (x+y=w327:dbl)
        }
        n117 = Bundle(w299, w297) -> (w293:cluster{dbl[], dbl[]})  [unwired: 1 in]
        n118 = Array Size(array=w304) -> (size(s)=w308:i32)
        n119 = Array Subset(array=w307, index=w309, length=w308) -> (w303:dbl[])
        n120 = Decimate 1D Array(w303) -> (w294:dbl[], w302:dbl[])
        n121 = Not A Number/Path/Refnum?(number/path/refnum=w294) -> (NaN/Path/Refnum?=w296:bool[])
        n122 = And Array Elements(Boolean array=w296) -> (logical AND=w295:bool)
        n123 = Bundle(w299, w294) -> (w301:cluster{dbl[], dbl[]})  [unwired: 1 in]
        n124 = Bundle(w299, w302) -> (w300:cluster{dbl[], dbl[]})  [unwired: 1 in]
        n125 = Build Array(w301, w300, w293) -> (w291:cluster{dbl[], dbl[]}[])
        n126 = case shown="True" w295 {
          tunnel: w293 -> [_ w324]
          tunnel: [w319 w323] -> w292
          tunnel: w291 -> [w319 _]
          frame False {
            n127 = property on="Panel Temps" class="XYGraph (strict)"("Active Plot"=u32 0, "Plot.Plot Name"="Dem Water Temp", "Active Plot"=u32 1, "Plot.Plot Name"="Y-ve Floor Water Return", "Active Plot"=u32 2, "Plot.Plot Name"="Y+ve Floor Water Return") -> ()  [unwired: 2 in, 2 out]
          }
          frame True {
            n128 = property on="Panel Temps" class="XYGraph (strict)"("Active Plot"=u32 0, "Plot.Plot Name"="Dem Water Temp") -> ()  [unwired: 2 in, 2 out]
            n129 = Build Array(w324) -> (w323:cluster{dbl[], dbl[]}[])
          }
        }
        n130 = Build Array (concatenate)(w310, w304) -> (w311:string[])
      }
      frame "Roof Panel Values" {
        w331 = string[] ["EnFlo_Tunnel:Temp:Roof_Far_2", "EnFlo_Tunnel:Temp:Roof_Near_3", "EnFlo_Tunnel:Temp:Roof_Far_4", "EnFlo_Tunnel:Temp:Roof_Far_6", "EnFlo_Tunnel:Temp:Roof_Near_7", "EnFlo_Tunnel:Temp:Roof_Far_8", "EnFlo_Tunnel:Temp:Roof_Far_10", "EnFlo_Tunnel:Temp:Roof_Near_12", "EnFlo_Tunnel:Temp:Roof_Far_15", "EnFlo_Tunnel:Temp:Roof_Far_19"] ("subarray")
        n131 = Array Size(array=w339) -> (size(s)=w338:i32)
        n132 = Array Size(array=w331) -> (size(s)=w337:i32)
        n133 = Array Subset(array=w336, index=w338, length=w337) -> (w332:dbl[])
        n134 = Build Array (concatenate)(w339, w331) -> (w340:string[])
        n135 = Bundle(dbl[] [1.5, 2.5, 3.5, 5.5, 6.5, 7.5, 9.5, 11.5, 14.5, 18.5], w332) -> (w329:cluster{dbl[], dbl[]})  [unwired: 1 in]
        n136 = Build Array (concatenate)(w334, w329) -> (w333:cluster{dbl[], dbl[]}[])
      }
      frame "Floor Surface Panels" {
        w344 = string[] ["EnFlo_Tunnel:Temp:Floor_Near_1", "EnFlo_Tunnel:Temp:Floor_Far_1", "EnFlo_Tunnel:Temp:Floor_2.1", "EnFlo_Tunnel:Temp:Floor_2.2", "EnFlo_Tunnel:Temp:Floor_2.3", "EnFlo_Tunnel:Temp:Floor_3.1", "EnFlo_Tunnel:Temp:Floor_3.2", "EnFlo_Tunnel:Temp:Floor_3.3", "EnFlo_Tunnel:Temp:Floor_4.1", "EnFlo_Tunnel:Temp:Floor_4.2", "EnFlo_Tunnel:Temp:Floor_4.3", "EnFlo_Tunnel:Temp:Floor_5.1", "EnFlo_Tunnel:Temp:Floor_5.2", "EnFlo_Tunnel:Temp:Floor_5.3", "EnFlo_Tunnel:Temp:Floor_6.1", "EnFlo_Tunnel:Temp:Floor_6.2", "EnFlo_Tunnel:Temp:Floor_6.3", "EnFlo_Tunnel:Temp:Floor_7.1", "EnFlo_Tunnel:Temp:Floor_7.2", "EnFlo_Tunnel:Temp:Floor_7.3", "EnFlo_Tunnel:Temp:Floor_8.1", "EnFlo_Tunnel:Temp:Floor_8.2", "EnFlo_Tunnel:Temp:Floor_8.3", "EnFlo_Tunnel:Temp:Floor_9.1", "EnFlo_Tunnel:Temp:Floor_9.2", "EnFlo_Tunnel:Temp:Floor_9.3", "EnFlo_Tunnel:Temp:Floor_10.1", "EnFlo_Tunnel:Temp:Floor_10.2", "EnFlo_Tunnel:Temp:Floor_10.3", "EnFlo_Tunnel:Temp:Floor_11.1", "EnFlo_Tunnel:Temp:Floor_11.2", "EnFlo_Tunnel:Temp:Floor_11.3", "EnFlo_Tunnel:Temp:Floor_12.1", "EnFlo_Tunnel:Temp:Floor_12.2", "EnFlo_Tunnel:Temp:Floor_12.3", "EnFlo_Tunnel:Temp:Floor_13.1", "EnFlo_Tunnel:Temp:Floor_13.2", "EnFlo_Tunnel:Temp:Floor_13.3", "EnFlo_Tunnel:Temp:Floor_14.1", "EnFlo_Tunnel:Temp:Floor_14.2", "EnFlo_Tunnel:Temp:Floor_14.3", "EnFlo_Tunnel:Temp:Floor_15.1", "EnFlo_Tunnel:Temp:Floor_15.2", "EnFlo_Tunnel:Temp:Floor_15.3", "EnFlo_Tunnel:Temp:Floor_16.1", "EnFlo_Tunnel:Temp:Floor_16.2", "EnFlo_Tunnel:Temp:Floor_16.3", "EnFlo_Tunnel:Temp:Floor_17.1", "EnFlo_Tunnel:Temp:Floor_17.2", "EnFlo_Tunnel:Temp:Floor_17.3", "EnFlo_Tunnel:Temp:Floor_18.1", "EnFlo_Tunnel:Temp:Floor_18.2", "EnFlo_Tunnel:Temp:Floor_18.3", "EnFlo_Tunnel:Temp:Floor_19.1", "EnFlo_Tunnel:Temp:Floor_19.2", "EnFlo_Tunnel:Temp:Floor_19.3"] ("subarray")
        n137 = Array Size(array=w353) -> (size(s)=w352:i32)
        n138 = Array Size(array=w344) -> (size(s)=w351:i32)
        n139 = Array Subset(array=w350, index=w352, length=w351) -> (w346:dbl[])
        n140 = Build Array (concatenate)(w353, w344) -> (w354:string[])
        n141 = Bundle("Array"=dbl[] [0.2, 0.6, 1.3, 1.6, 1.9, 2.3, 2.6, 2.9, 3.3, 3.6, 3.9, 4.3, 4.6, 4.9, 5.3, 5.6, 5.9, 6.3, 6.6, 6.9, 7.3, 7.6, 7.9, 8.3, 8.6, 8.9, 9.3, 9.6, 9.9, 10.3, 10.6, 10.9, 11.3, 11.6, 11.9, 12.3, 12.6, 12.9, 13.3, 13.6, 13.9, 14.3, 14.6, 14.9, 15.3, 15.6, 15.9, 16.3, 16.6, 16.9, 17.3, 17.6, 17.9, 18.3, 18.6, 18.9], w346) -> (w345:cluster{"Array":dbl[], dbl[]})  [unwired: 1 in]
        n142 = Build Array (concatenate)(w348, w345) -> (w347:cluster{"Array":dbl[], dbl[]}[])
      }
      frame "Floor Panel Averages" {
        w357 = string[] ["EnFlo_Tunnel:Temp:Floor_Near_1", "EnFlo_Tunnel:Temp:Floor_Far_1", "EnFlo_Tunnel:Temp:Floor_2", "EnFlo_Tunnel:Temp:Floor_3", "EnFlo_Tunnel:Temp:Floor_4", "EnFlo_Tunnel:Temp:Floor_5", "EnFlo_Tunnel:Temp:Floor_6", "EnFlo_Tunnel:Temp:Floor_7", "EnFlo_Tunnel:Temp:Floor_8", "EnFlo_Tunnel:Temp:Floor_9", "EnFlo_Tunnel:Temp:Floor_10", "EnFlo_Tunnel:Temp:Floor_11", "EnFlo_Tunnel:Temp:Floor_12", "EnFlo_Tunnel:Temp:Floor_13", "EnFlo_Tunnel:Temp:Floor_14", "EnFlo_Tunnel:Temp:Floor_15", "EnFlo_Tunnel:Temp:Floor_16", "EnFlo_Tunnel:Temp:Floor_17", "EnFlo_Tunnel:Temp:Floor_18", "EnFlo_Tunnel:Temp:Floor_19"] ("subarray")
        n143 = Array Size(array=w367) -> (size(s)=w366:i32)
        n144 = Array Size(array=w357) -> (size(s)=w365:i32)
        n145 = Array Subset(array=w364, index=w366, length=w365) -> (w360:dbl[])
        n146 = Build Array (concatenate)(w367, w357) -> (w368:string[])
        n147 = Bundle("Array"=dbl[] [0.3, 0.6, 1.5, 2.5, 3.5, 4.5, 5.5, 6.5, 7.5, 8.5, 9.5, 10.5, 11.5, 12.5, 13.5, 14.5, 15.5, 16.5, 17.5, 18.5], w360) -> (w359:cluster{"Array":dbl[], dbl[]})  [unwired: 1 in]
        n148 = Build Array (concatenate)(w362, w359) -> (w361:cluster{"Array":dbl[], dbl[]}[])
      }
      frame "Floor Panel Setpoints" {
        w372 = string[] ["EnFlo_Tunnel:Setpoint:Floor_Far_1", "EnFlo_Tunnel:Setpoint:Floor_Near_1", "EnFlo_Tunnel:Setpoint:Floor_2", "EnFlo_Tunnel:Setpoint:Floor_3", "EnFlo_Tunnel:Setpoint:Floor_4", "EnFlo_Tunnel:Setpoint:Floor_5", "EnFlo_Tunnel:Setpoint:Floor_6", "EnFlo_Tunnel:Setpoint:Floor_7", "EnFlo_Tunnel:Setpoint:Floor_8", "EnFlo_Tunnel:Setpoint:Floor_9", "EnFlo_Tunnel:Setpoint:Floor_10", "EnFlo_Tunnel:Setpoint:Floor_11", "EnFlo_Tunnel:Setpoint:Floor_12", "EnFlo_Tunnel:Setpoint:Floor_13", "EnFlo_Tunnel:Setpoint:Floor_14", "EnFlo_Tunnel:Setpoint:Floor_15", "EnFlo_Tunnel:Setpoint:Floor_16", "EnFlo_Tunnel:Setpoint:Floor_17", "EnFlo_Tunnel:Setpoint:Floor_18", "EnFlo_Tunnel:Setpoint:Floor_19"] ("subarray")
        n149 = Array Size(array=w381) -> (size(s)=w380:i32)
        n150 = Array Size(array=w372) -> (size(s)=w379:i32)
        n151 = Array Subset(array=w378, index=w380, length=w379) -> (w374:dbl[])
        n152 = Build Array (concatenate)(w381, w372) -> (w382:string[])
        n153 = Bundle("Array"=dbl[] [0.3, 0.6, 1.5, 2.5, 3.5, 4.5, 5.5, 6.5, 7.5, 8.5, 9.5, 10.5, 11.5, 12.5, 13.5, 14.5, 15.5, 16.5, 17.5, 18.5], w374) -> (w373:cluster{"Array":dbl[], dbl[]})  [unwired: 1 in]
        n154 = Build Array (concatenate)(w376, w373) -> (w375:cluster{"Array":dbl[], dbl[]}[])
      }
      frame "Floor Panel Powers" {
        w387 = string[] ["EnFlo_Tunnel:Power:Floor_Up_Y=-1585", "EnFlo_Tunnel:Power:Floor_Up_Y=-1250", "EnFlo_Tunnel:Power:Floor_Up_Y=-920", "EnFlo_Tunnel:Power:Floor_Up_Y=-585", "EnFlo_Tunnel:Power:Floor_Up_Y=-250", "EnFlo_Tunnel:Power:Floor_Up_Y=80", "EnFlo_Tunnel:Power:Floor_Up_Y=415", "EnFlo_Tunnel:Power:Floor_Up_Y=750", "EnFlo_Tunnel:Power:Floor_Up_Y=1080", "EnFlo_Tunnel:Power:Floor_Up_Y=1415", "EnFlo_Tunnel:Power:Floor_Down_Y=-1250", "EnFlo_Tunnel:Power:Floor_Down_Y=-920", "EnFlo_Tunnel:Power:Floor_Down_Y=-585", "EnFlo_Tunnel:Power:Floor_Down_Y=-250", "EnFlo_Tunnel:Power:Floor_Down_Y=80", "EnFlo_Tunnel:Power:Floor_Down_Y=415", "EnFlo_Tunnel:Power:Floor_Down_Y=750", "EnFlo_Tunnel:Power:Floor_Down_Y=1080"] ("subarray")
        n155 = Array Size(array=w394) -> (size(s)=w393:i32)
        n156 = Array Size(array=w387) -> (size(s)=w392:i32)
        n157 = Array Subset(array=w391, index=w393, length=w392) -> (w389:dbl[])
        n158 = Build Array (concatenate)(w394, w387) -> (w395:string[])
        n159 = Bundle("Array"=dbl[] [-1585.0, -1250.0, -920.0, -585.0, -250.0, 80.0, 415.0, 750.0, 1080.0, 1415.0, -1250.0, -920.0, -585.0, -250.0, 80.0, 415.0, 750.0, 1080.0], w389) -> (→"Floor Powers":cluster{"Array":dbl[], dbl[]})  [unwired: 1 in]
      }
      frame "Lab Stratification" {
        w412 = dbl[] [0.0, 6.0]
        w415 = 8 ("length")
        w427 = dbl[] [5.75, 4.5, 3.5, 2.5, 1.5, 0.5, 0.1, 0.0]
        n160 = Array Size(array=w430) -> (size(s)=w414:i32)
        n161 = Add(x=w414, y=w415) -> (x+y=w413:i32)
        n162 = Array Subset(array=w417, index=w413) -> (w416:dbl[])  [unwired: 1 in]
        n163 = Index Array(array=w416) -> (element #1=→"Delta T":dbl, element #2=w409:dbl, element #3=→"Heat Extraction kW":dbl, element #4=w411:dbl)  [unwired: 4 in]
        "Av Lab Temp" <- w409
        "Des Air Temp" <- w411
        n164 = Array Subset(array=w417, index=w414, length=w415) -> (w420:dbl[])
        n165 = for {
          N: 15 -> [_]
          tunnel: 2.43 -> [w437]
          tunnel: [w435] -> w424 mode=indexing
          i -> [w439]
          n166 = Multiply(x=0.1, y=w439) -> (x*y=w436:dbl)
          n167 = Subtract(x=w437, y=w436) -> (x-y=w435:dbl)
        }
        n168 = call <vilib>:"Interpolate 1D.vi"("xi"=w424, "X"=w427, "Y"=w420) -> ("yi"=w423:dbl[])  [unwired: 3 in, 5 out]
        n169 = Build Array(w411, w411) -> (w410:dbl[])
        n170 = Build Array(w409, w409) -> (w408:dbl[])
        n171 = local read "Heaters Enabled"() -> (w399:bool)
        n172 = Bundle(w420, w427) -> (w407:cluster{dbl[], dbl[]})  [unwired: 1 in]
        n173 = Bundle(w410, w412) -> (w406:cluster{dbl[], dbl[]})  [unwired: 1 in]
        n174 = Bundle(w408, w412) -> (w405:cluster{dbl[], dbl[]})  [unwired: 1 in]
        n175 = Bundle("yi"=w423, w403) -> (w422:cluster{"yi":dbl[], dbl[]})  [unwired: 1 in]
        n176 = case shown="False" w399 {
          tunnel: ["Get Server Values" "Inlet Heater Setpoint Values"] -> w398
          frame False {
          }
          frame True {
          }
        }
        n177 = Build Array(w407, w406, w405) -> (→"Strat":cluster{dbl[], dbl[]}[])
        n178 = Build Array (concatenate)(w430, string[] ["EnFlo Lab:labstrat1:Z=5.75m Roof", "EnFlo Lab:labstrat1:Z=4.5m", "EnFlo Lab:labstrat1:Z=3.5m", "EnFlo Lab:labstrat1:Z=2.5m", "EnFlo Lab:labstrat1:Z=1.5m", "EnFlo Lab:labstrat1:Z=0.5m", "EnFlo Lab:labstrat1:Z=0.1m", "EnFlo Lab:labstrat1:Z=0m Floor", "EnFlo Lab:labstrat1:Delta T", "EnFlo Lab:labstrat1:Av Temp", "EnFlo Lab:Heat:Extraction", "EnFlo Lab:Desired:Air Temp"] ("subarray")) -> (w431:string[])
        n179 = Array Size(array=w400) -> (size(s)=w401:i32)
        n180 = Build Array (concatenate)(w400, w422) -> (w421:cluster{"yi":dbl[], dbl[]}[])
        n181 = property on="Inlet Heaters" class="XYGraph (strict)"("Active Plot"=w401, "Plot.Plot Name"="Lab Strat") -> ()  [unwired: 2 in, 2 out]
      }
      frame "Inlet Heater Setpoint Values" {
        w440 = string[] ["EnFlo_Tunnel:Setpoint:Inlet_Y=0_Z=1450", "EnFlo_Tunnel:Setpoint:Inlet_Y=0_Z=1350", "EnFlo_Tunnel:Setpoint:Inlet_Y=0_Z=1250", "EnFlo_Tunnel:Setpoint:Inlet_Y=0_Z=1150", "EnFlo_Tunnel:Setpoint:Inlet_Y=0_Z=1050", "EnFlo_Tunnel:Setpoint:Inlet_Y=0_Z=950", "EnFlo_Tunnel:Setpoint:Inlet_Y=0_Z=850", "EnFlo_Tunnel:Setpoint:Inlet_Y=0_Z=750", "EnFlo_Tunnel:Setpoint:Inlet_Y=0_Z=650", "EnFlo_Tunnel:Setpoint:Inlet_Y=0_Z=550", "EnFlo_Tunnel:Setpoint:Inlet_Y=0_Z=450", "EnFlo_Tunnel:Setpoint:Inlet_Y=0_Z=350", "EnFlo_Tunnel:Setpoint:Inlet_Y=0_Z=250", "EnFlo_Tunnel:Setpoint:Inlet_Y=0_Z=150", "EnFlo_Tunnel:Setpoint:Inlet_Y=0_Z=50"] ("subarray")
        n182 = Array Size(array=w455) -> (size(s)=w454:i32)
        n183 = Array Size(array=w443) -> (size(s)=w441:i32)
        n184 = property on="Inlet Heaters" class="XYGraph (strict)"("Active Plot"=w441, "Plot.Plot Name"="Inlet Setpoints") -> ()  [unwired: 2 in, 2 out]
        n185 = Array Size(array=w440) -> (size(s)=w453:i32)
        n186 = Array Subset(array=w452, index=w454, length=w453) -> (w445:dbl[])
        n187 = Bundle(w445, w444) -> (w451:cluster{dbl[], dbl[]})  [unwired: 1 in]
        n188 = for {
          tunnel: i32[] [14, 10, 5, 0] -> [w460] mode=indexing
          tunnel: w445 -> [w458]
          tunnel: [w459] -> w447 mode=indexing
          n189 = Index Array(array=w458, index=w460) -> (element=w459:dbl)
        }
        "Setpoints" <- w447
        n190 = Build Array (concatenate)(w455, w440) -> (w456:string[])
        n191 = Build Array (concatenate)(w443, w451) -> (w450:cluster{"yi":dbl[], dbl[]}[])
      }
      frame "Inlet Heater Power Values" {
        w461 = string[] ["EnFlo_Tunnel:Power:Inlet_Y=0_Z=1450", "EnFlo_Tunnel:Power:Inlet_Y=0_Z=1350", "EnFlo_Tunnel:Power:Inlet_Y=0_Z=1250", "EnFlo_Tunnel:Power:Inlet_Y=0_Z=1150", "EnFlo_Tunnel:Power:Inlet_Y=0_Z=1050", "EnFlo_Tunnel:Power:Inlet_Y=0_Z=950", "EnFlo_Tunnel:Power:Inlet_Y=0_Z=850", "EnFlo_Tunnel:Power:Inlet_Y=0_Z=750", "EnFlo_Tunnel:Power:Inlet_Y=0_Z=650", "EnFlo_Tunnel:Power:Inlet_Y=0_Z=550", "EnFlo_Tunnel:Power:Inlet_Y=0_Z=450", "EnFlo_Tunnel:Power:Inlet_Y=0_Z=350", "EnFlo_Tunnel:Power:Inlet_Y=0_Z=250", "EnFlo_Tunnel:Power:Inlet_Y=0_Z=150", "EnFlo_Tunnel:Power:Inlet_Y=0_Z=50"] ("subarray")
        n192 = Array Size(array=w474) -> (size(s)=w473:i32)
        n193 = Array Size(array=w463) -> (size(s)=w464:i32)
        n194 = Array Size(array=w461) -> (size(s)=w472:i32)
        n195 = Array Subset(array=w471, index=w473, length=w472) -> (w470:dbl[])
        n196 = Bundle(w470, w468) -> (w466:cluster{dbl[], dbl[]})  [unwired: 1 in]
        n197 = Build Array (concatenate)(w474, w461) -> (w475:string[])
        n198 = property on="Inlet Heaters" class="XYGraph (strict)"("Active Plot"=w464, "Plot.Plot Name"="Inlet Powers") -> ()  [unwired: 2 in, 2 out]
        n199 = Build Array (concatenate)(w463, w466) -> (w467:cluster{"yi":dbl[], dbl[]}[])
      }
      frame "Power Y=-1500" {
        w477 = string[] ["EnFlo_Tunnel:Power:Inlet_Y=-1500_Z=1450", "EnFlo_Tunnel:Power:Inlet_Y=-1500_Z=1350", "EnFlo_Tunnel:Power:Inlet_Y=-1500_Z=1250", "EnFlo_Tunnel:Power:Inlet_Y=-1500_Z=1150", "EnFlo_Tunnel:Power:Inlet_Y=-1500_Z=1050", "EnFlo_Tunnel:Power:Inlet_Y=-1500_Z=950", "EnFlo_Tunnel:Power:Inlet_Y=-1500_Z=850", "EnFlo_Tunnel:Power:Inlet_Y=-1500_Z=750", "EnFlo_Tunnel:Power:Inlet_Y=-1500_Z=650", "EnFlo_Tunnel:Power:Inlet_Y=-1500_Z=550", "EnFlo_Tunnel:Power:Inlet_Y=-1500_Z=450", "EnFlo_Tunnel:Power:Inlet_Y=-1500_Z=350", "EnFlo_Tunnel:Power:Inlet_Y=-1500_Z=250", "EnFlo_Tunnel:Power:Inlet_Y=-1500_Z=150", "EnFlo_Tunnel:Power:Inlet_Y=-1500_Z=50"] ("subarray")
        n200 = Array Size(array=w490) -> (size(s)=w489:i32)
        n201 = Array Size(array=w479) -> (size(s)=w480:i32)
        n202 = Array Size(array=w477) -> (size(s)=w488:i32)
        n203 = Array Subset(array=w487, index=w489, length=w488) -> (w486:dbl[])
        n204 = Bundle(w486, w484) -> (w482:cluster{dbl[], dbl[]})  [unwired: 1 in]
        n205 = Build Array (concatenate)(w490, w477) -> (w491:string[])
        n206 = property on="Inlet Heaters" class="XYGraph (strict)"("Active Plot"=w480, "Plot.Plot Name"="Power Y=-1500") -> ()  [unwired: 2 in, 2 out]
        n207 = Build Array (concatenate)(w479, w482) -> (w483:cluster{"yi":dbl[], dbl[]}[])
      }
      frame "Get Server Values" {
        n208 = Multiply(x="History in Minutes", y=60.0) -> (x*y=w495:dbl)
        n209 = call "Get_Channel_averages.vi"("Desired Ch Names"=w504, "Averaging time (mins)"="Averaging time (mins)", "End Offset Sec (0)"=w495) -> ("number"=w503:dbl[])  [unwired: 2 out]
        n210 = Not(x="Stop Button") -> (.not. x?=w500:bool)
      }
    }
  }
